vi "PFI-28000-Card-28144_Get Fault Scan Enable.vi"(8 "error in (no error)":errorcluster, 11 "PFI-28000-Card-28144 in":refnum<class "PFI-28000-Card-28144.lvclass">) -> (0 "error out":errorcluster, 2 "Enable":bool, 3 "PFI-28000-Card-28144 out":refnum<class "PFI-28000-Card-28144.lvclass">)   [LabVIEW 2017, in "PFI-28000-Card-28144.lvclass"]
uses:
  PFI-28000-Card-28144.lvclass
  C:/wc/07143 Precision Filters 28000 Support/Driver/source/Card/PFI-28000-Card.lvclass
  Channel/PFI-28000-Channel.lvclass
  Utilities/PFI-28000-Utils.lvlib
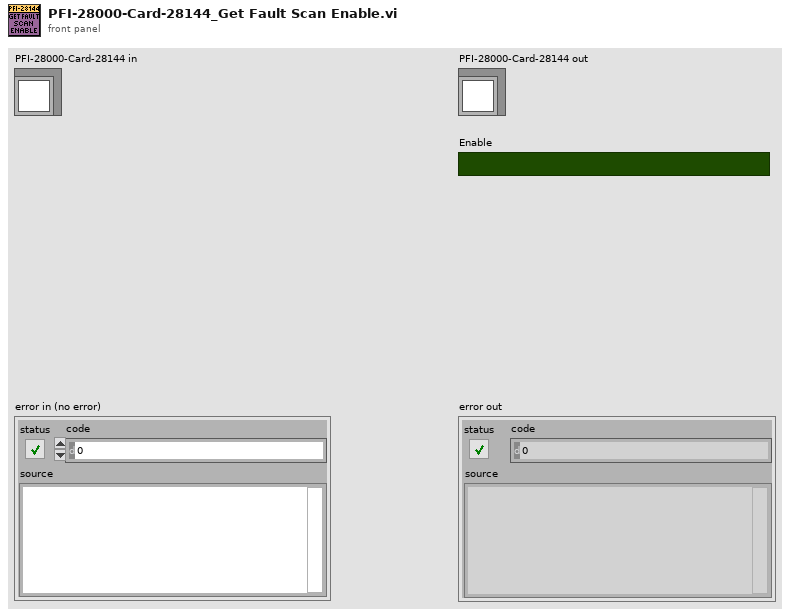
[diagram p1: front panel]
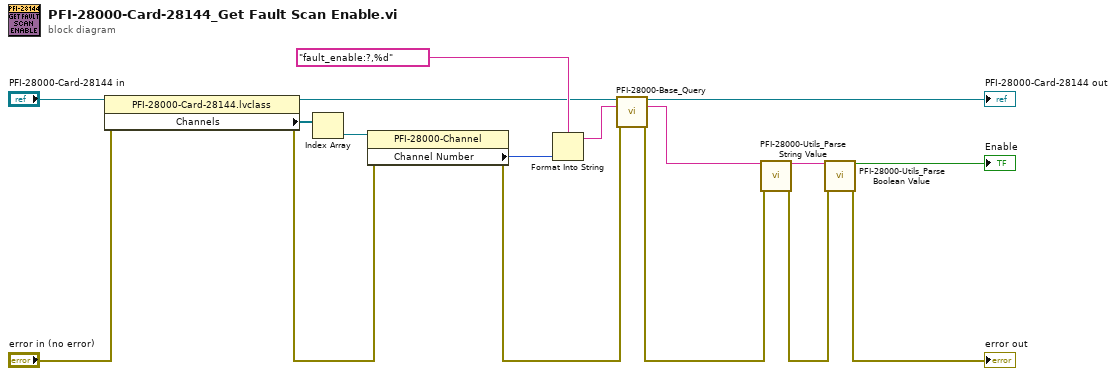
[diagram p0: block diagram]
diagram:
  n1 = property class="PFI-28000-Card-28144.lvclass"(reference="PFI-28000-Card-28144 in", error in="error in (no error)") -> (reference out=w6:refnum<class "PFI-28000-Card-28144.lvclass">, error out=w14:errorcluster, "Channels"=w13:refnum<class "PFI-28000-Channel.lvclass">[])
  n2 = Index Array(array=w13) -> (element=w12:refnum<class "PFI-28000-Channel.lvclass">)  [unwired: 1 in]
  n3 = property class="PFI-28000-Channel"(reference=w12, error in=w14) -> (error out=w4:errorcluster, "Channel Number"=w11:i32)  [unwired: 1 out]
  n4 = Format Into String(format string="fault_enable:?,%d" ("empty string"), w11) -> (resulting string=w5:string)  [unwired: 2 in, 1 out]
  n5 = call-dynamic "PFI-28000-Base_Query.vi"("PFI-28000-Base in"=w6, "Command"=w5, "error in (no error)"=w4) -> ("PFI-28000-Base out"=→"PFI-28000-Card-28144 out":refnum<class "PFI-28000-Card-28144.lvclass">, "Response"=w2:string, "error out"=w3:errorcluster)  [unwired: 9 in, 1 out]
  n6 = call "PFI-28000-Utils_Parse String Value.vi"("String"=w2, "error in (no error)"=w3) -> ("String Value"=w10:string, "error out"=w9:errorcluster)  [unwired: 11 in, 1 out]
  n7 = call "PFI-28000-Utils_Parse Boolean Value.vi"("String"=w10, "error in (no error)"=w9) -> ("Value"=→"Enable":bool, "error out"=→"error out":errorcluster)  [unwired: 12 in]
